vi "PAN_FinishCallback.vi"(5 "wait":bool=TRUE, 6 "obsID":string, 8 "error in (no error)":errorcluster, 9 "Command":string, 10 "response in":string) -> (2 "response out":string)   [LabVIEW 2016]
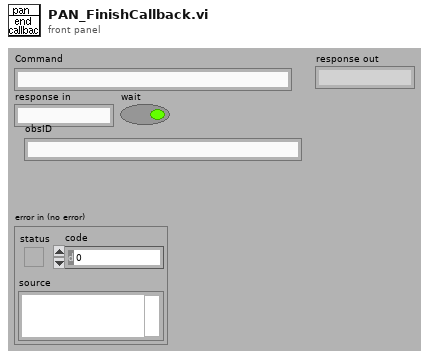
[diagram p1: front panel]
types:
  T1 = enum16{"add", "delete", "clean", "shutdown", "hold", "continue", "modify"}
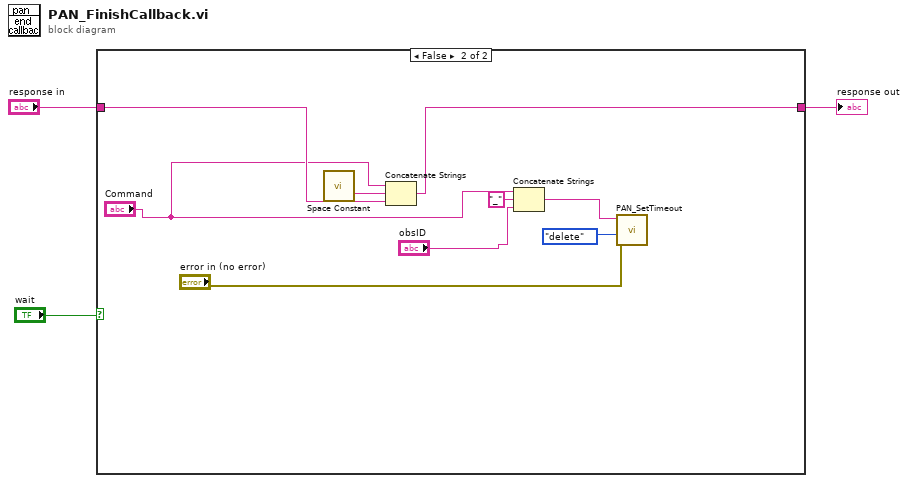
[diagram p0: block diagram]
diagram:
  n1 = case shown="False" "wait" {
    tunnel: "response in" -> [w4 w10]
    tunnel: [w4 w9] -> w1
    frame True {
    }
    frame False {
      n2 = call <vilib>:"Space Constant.vi"() -> ("String"=w11:string)
      n3 = Concatenate Strings("Command", w11, w10) -> (w9:string)
      n4 = Concatenate Strings("Command", "_" ("string"), "obsID") -> (w5:string)
      n5 = call "PAN_SetTimeout.vi"("error in (no error)"="error in (no error)", "action"=T1."delete", "Command"=w5) -> ()  [unwired: 1 in, 8 out]
    }
  }
  "response out" <- w1
